vi "Save Settings to XML.vi"(8 "error in (no error)":errorcluster, 11 "Settings":T1={"Hardware Configuration"={"VISA resource name"="", "DAQ Type"=enum."Simulated", "Channel 1"={"Acquiring"=FALSE, "Enabled"=FALSE, "Terminal configuration"=0, "Range"=0}, "Channel 2"={"Acquiring"=FALSE, "Enabled"=FALSE, "Terminal configuration"=0, "Range"=0}, "Timing"={"Sample Rate"=0, "Actual Sample Rate"=0, "Samples per Iteration"=0, "Sample Clock Source"=0, "Time Units"=0}, "PS Parameters"={"PS handle"=0, "PS Max_adc"=32767, "PS Enabled Array"=[], "PS Device Info"={"Driver Version"="", "USB Version"="", "Hardware"="", "Variant"="", "Batch and Serial"="", "Cal Date"="", "Kernel Version"="", "Digital HW Version"="", "Analogue HW Version"="", "Firmware 1"="", "Firmware 2"="", "MSO"=FALSE, "Number of Channels"=0}, "Channel 1 Buffer"=refnum, "Channel 2 Buffer"=refnum}, "Trigger"={"Trigger Source"=0, "Direction"=0, "Threshold [V]"=0.0, "Enabled"=FALSE}, "Keithley Parameters"={"Previous End / Current Start"=0}}, "Logging Configuration"={"Log File Base Path"=path "", "TDMS File Reference"=refnum, "Enabled"=FALSE}} {"Hardware Configuration"."Trigger"."Direction" items=["Falling", "Rising"]; "Hardware Configuration"."Trigger"."Trigger Source" items=["Channel 1", "Channel 2", "External"]; "Hardware Configuration"."Timing"."Time Units" items=["Seconds"]; "Hardware Configuration"."Timing"."Sample Clock Source" items=["Internal", "External"]; "Hardware Configuration"."Channel 2"."Terminal configuration" items=["Referenced Single Ended", "Differential"]; "Hardware Configuration"."Channel 1"."Terminal configuration" items=["Referenced Single Ended", "Differential"]}) -> (0 "error out":errorcluster)   [LabVIEW 2016, in "Settings.lvlib"]
doc: "Saves the \"User Specified\" configuration data to an XML file. This is used to remember the users settings between executions."
uses:
  Settings.lvlib
  Settings.ctl
  Acquisition/Hardware Configuration.ctl
  Acquisition/Signal Type.ctl
  Logging/Logging Configuration.ctl
  <vilib>/Utility/xml.llb/Write to XML File(string).vi
  Acquisition/Acquisition.lvlib
  Logging/Logging.lvlib
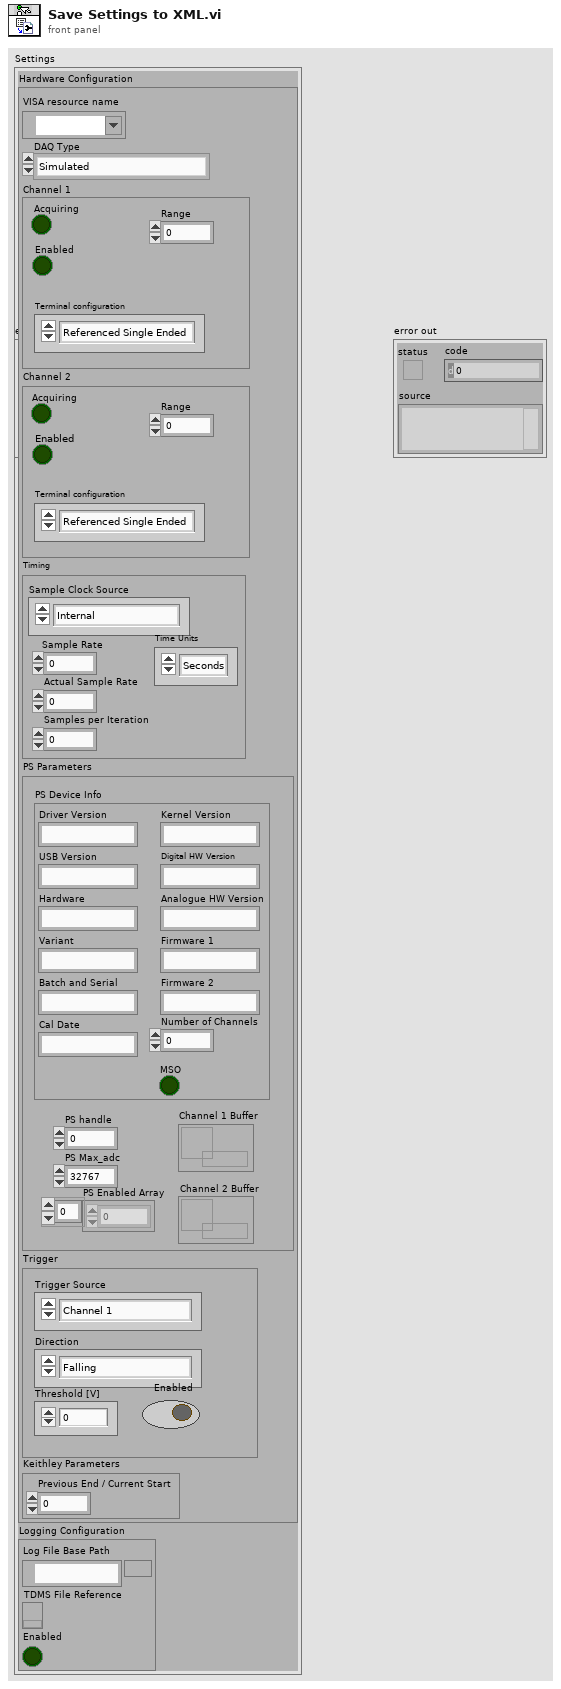
[diagram p1: front panel]
types:
  T1 = typedef "Settings.lvlib/Settings.ctl" = cluster{"Hardware Configuration":T2, "Logging Configuration":T4}
  T2 = typedef "Acquisition.lvlib/Hardware Configuration.ctl" = cluster{"VISA resource name":refnum<visa-resource-name>, "DAQ Type":T3, "Channel 1":cluster{"Acquiring":bool, "Enabled":bool, "Terminal configuration":u16, "Range":u16}, "Channel 2":cluster{"Acquiring":bool, "Enabled":bool, "Terminal configuration":u16, "Range":u16}, "Timing":cluster{"Sample Rate":u32, "Actual Sample Rate":u32, "Samples per Iteration":u32, "Sample Clock Source":u16, "Time Units":u16}, "PS Parameters":cluster{"PS handle":i16, "PS Max_adc":i16, "PS Enabled Array":i16[], "PS Device Info":cluster{"Driver Version":string, "USB Version":string, "Hardware":string, "Variant":string, "Batch and Serial":string, "Cal Date":string, "Kernel Version":string, "Digital HW Version":string, "Analogue HW Version":string, "Firmware 1":string, "Firmware 2":string, "MSO":bool, "Number of Channels":i16}, "Channel 1 Buffer":refnum<data-value>, "Channel 2 Buffer":refnum<data-value>}, "Trigger":cluster{"Trigger Source":u16, "Direction":u16, "Threshold [V]":dbl, "Enabled":bool}, "Keithley Parameters":cluster{"Previous End / Current Start":i32}}
  T3 = typedef "Acquisition.lvlib/Signal Type.ctl" = enum16{"Simulated", "Tektronics DPO2k/3k/4k", "PicoScope 2000a Series", "Keithley DMM7510", "PicoScope 5000a Series"}
  T4 = typedef "Logging.lvlib/Logging Configuration.ctl" = cluster{"Log File Base Path":path, "TDMS File Reference":refnum<k34>, "Enabled":bool}
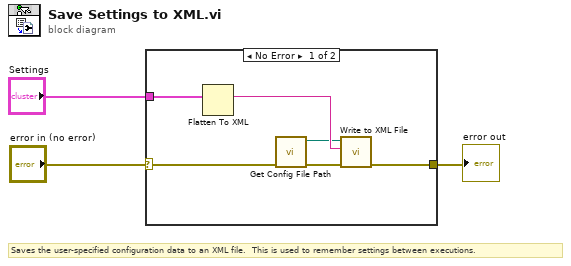
[diagram p0: block diagram]
diagram:
  # "Saves the user-specified configuration data to an XML file.  This is used to remember settings between executions."
  n1 = case shown="No Error" "error in (no error)" {
    selector: "error in (no error)" -> [w5 w10]
    tunnel: [w7 w10] -> w2
    tunnel: "Settings" -> [w9 _]
    frame No Error {
      n2 = Flatten To XML(anything=w9) -> (xml string=w8:string)
      n3 = call "Get Config File Path.vi"("error in (no error)"=w5) -> ("error out"=w4:errorcluster, "XML File Path"=w6:path)  [unwired: 9 in]
      n4 = call-poly <vilib>:"Write to XML File.vi"("error in (no error)"=w4, "XML Input"=w8, "XML File Path"=w6) -> ("error out"=w7:errorcluster)  [unwired: 6 in, 2 out]
    }
    frame Error {
    }
  }
  "error out" <- w2
